vi "Set Items (Label).vi"(6 "Items":refnum<class "IObject.lvclass">[](array[class]), 8 "error in (no error)":errorcluster, 10 "Label":string, 11 "MMI Scaling in":refnum<class "Interaction By Refererence.lvclass">) -> (0 "error out":errorcluster, 2 "Match?":bool, 3 "MMI Scaling out":refnum<class "Interaction By Refererence.lvclass">, 5 "Old items":refnum<class "IObject.lvclass">[](array[class]))   [LabVIEW 2021, in "Interaction By Refererence.lvclass"]
uses:
  Interaction By Refererence.lvclass
  IObject.lvclass
  Interaction By Refererence.lvclass/Interaction By Refererence.ctl
  IContainer/Interaction/Interaction.lvclass
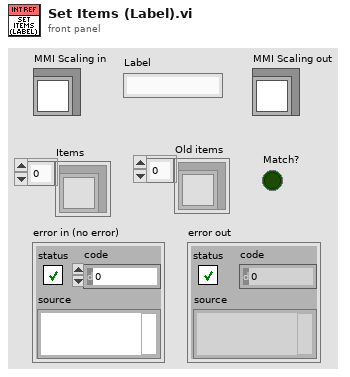
[diagram p1: front panel]
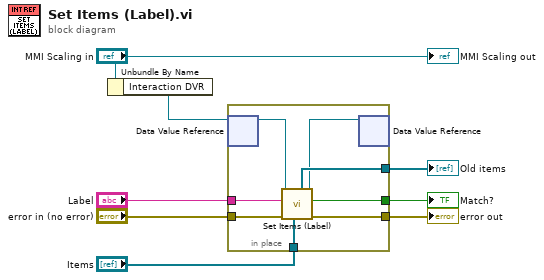
[diagram p0: block diagram]
diagram:
  n1 = Unbundle By Name("MMI Scaling in") -> ("Interaction DVR"=w1:refnum<data-value>)
  n2 = in-place {
    in-place-border: [w16] -> w8
    in-place-border: [w15] -> w7
    in-place-border: [w14] -> w6
    in-place-border: "Items" -> [w13]
    in-place-border: "error in (no error)" -> [w12]
    in-place-border: "Label" -> [w11]
    n3 = in-place-dvr #1(w1) -> (w10:refnum<class "Interaction.lvclass">)  [unwired: 1 out]
    n4 = call-dynamic "Set Items (Label).vi"("Items"=w13, "error in (no error)"=w12, "Label"=w11, "MMI Scaling in"=w10) -> ("error out"=w16:errorcluster, "Match?"=w15:bool, "MMI Scaling out"=w9:refnum<class "Interaction.lvclass">, "Old items"=w14:refnum<class "IObject.lvclass">[])  [unwired: 4 in]
    n5 = in-place-dvr #1(w9) -> ()  [unwired: 2 out]
  }
  "error out" <- w8
  "Match?" <- w7
  "Old items" <- w6
  "MMI Scaling out" <- "MMI Scaling in"
